vi "Refresh Access Codes.vi"(8 "error in":errorcluster, 9 "Refresh Token In":string, 11 "Authorization Code In":string) -> (0 "error out":errorcluster, 1 "Cluster":T1)   [LabVIEW 2016]
uses:
  <vilib>/httpClient/POSTBuffer.vi
  <vilib>/addons/_JKI.lib/Serialization/JSON/JKI JSON Serialization.lvlib
  <vilib>/httpClient/LabVIEWHTTPClient.lvlib
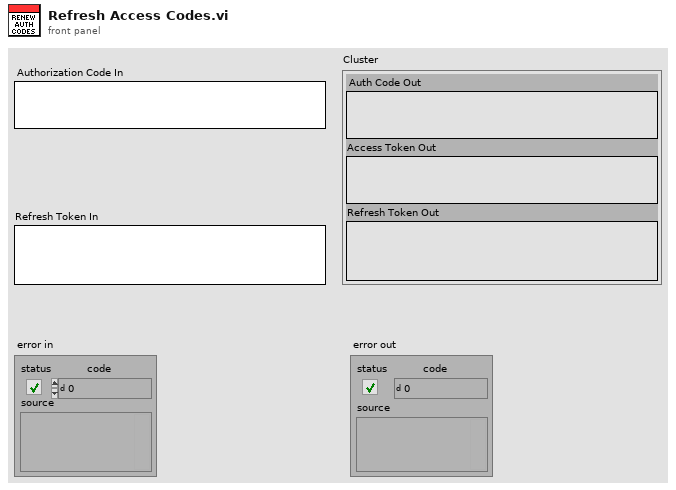
[diagram p1: front panel]
types:
  T1 = cluster{"Auth Code Out":string, "Access Token Out":string, "Refresh Token Out":string}
  T2 = cluster{"Access":string, "Refresh":string, "Authentication":string}
  T3 = cluster{"token_type":string, "scope":string, "access_token":string, "refresh_token":string, "user_id":string, "expires_in":i32}
  T4 = typedef "LabVIEWHTTPClient.lvlib/ClientHandle.ctl" = refnum<k1>
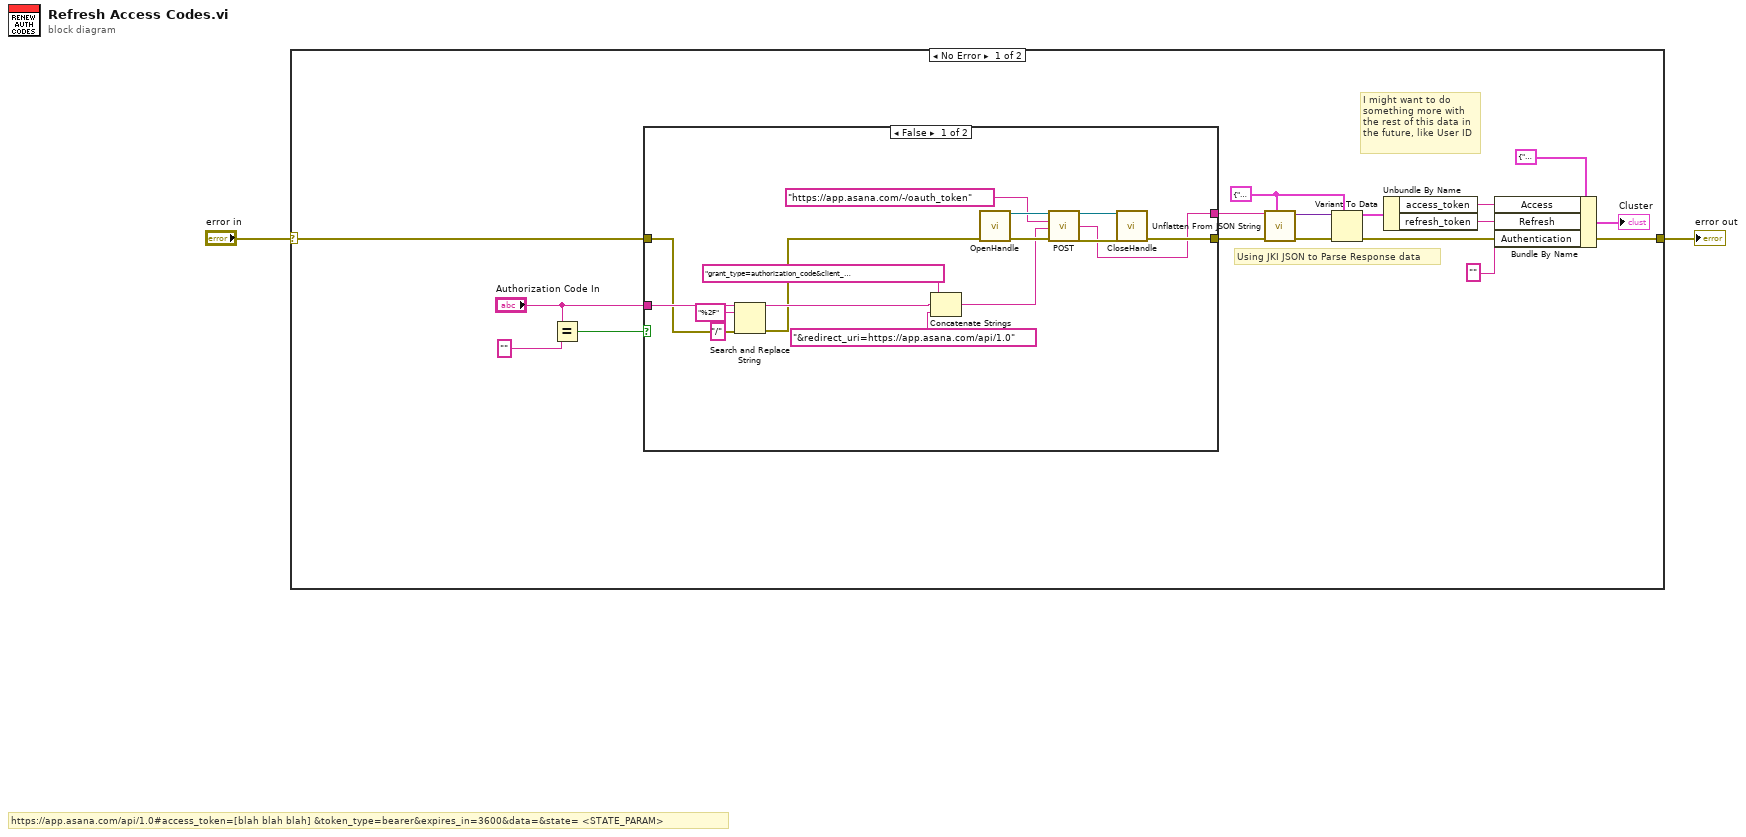
[diagram p0: block diagram]
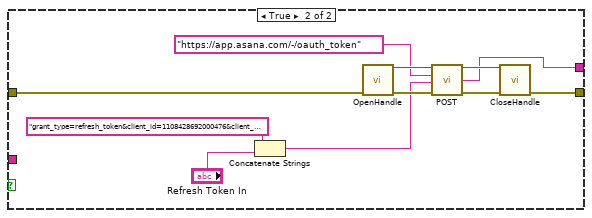
[diagram p2: hidden frame]
diagram:
  # "https://app.asana.com/api/1.0#access_token=[blah blah blah] &token_type=bearer&expires_in=3600&data=&state= <STATE_PARAM>"
  n1 = case shown="No Error" "error in" {
    selector: "error in" -> [w11 w46]
    tunnel: [w18 w46] -> w1
    frame No Error {
      w16 = T3 {"token_type"="", "scope"="", "access_token"="", "refresh_token"="", "user_id"="", "expires_in"=0}
      # "I might want to do something more with the rest of this data in the future, like User ID"
      # "Using JKI JSON to Parse Response data"
      n2 = Equal?(x="Authorization Code In", y="") -> (x = y?=w13:bool)
      n3 = case shown="False" w13 {
        tunnel: w11 -> [w22 w38]
        tunnel: [w31 w35] -> w10
        tunnel: [w25 w36] -> w8
        tunnel: "Authorization Code In" -> [w24 _]
        frame False {
          n4 = Search and Replace String(input string=w24, search string="%2F", replace string="/" ("replace string (\"\")"), error in=w22) -> (result string=w23:string, error out=w21:errorcluster)  [unwired: 4 in, 2 out]
          n5 = Concatenate Strings("grant_type=authorization_code&client_id=1108428692000476&client_secret=803bdca1138fccb00921b8f346728904&code=", w23, "&redirect_uri=https://app.asana.com/api/1.0") -> (w27:string)
          n6 = call <vilib>:"OpenHandle.vi"("error in (no error)"=w21) -> ("client handle out"=w30:T4, "error out"=w33:errorcluster)  [unwired: 13 in]
          n7 = call-poly <vilib>:"POST.vi"("client handle"=w30, "url"="https://app.asana.com/-/oauth_token", "buffer"=w27, "error in (no error)"=w33) -> ("client handle out"=w29:T4, "body"=w25:string, "error out"=w32:errorcluster)  [unwired: 8 in, 1 out]
          n8 = call <vilib>:"CloseHandle.vi"("client handle"=w29, "error in (no error)"=w32) -> ("error out"=w31:errorcluster)  [unwired: 13 in]
        }
        frame True {
          n9 = Concatenate Strings("grant_type=refresh_token&client_id=1108428692000476&client_secret=803bdca1138fccb00921b8f346728904&redirect_uri=https://app.asana.com/api/1.0&refresh_token=", "Refresh Token In") -> (w37:string)
          n10 = call <vilib>:"OpenHandle.vi"("error in (no error)"=w38) -> ("client handle out"=w41:T4, "error out"=w43:errorcluster)  [unwired: 13 in]
          n11 = call-poly <vilib>:"POST.vi"("client handle"=w41, "url"="https://app.asana.com/-/oauth_token", "buffer"=w37, "error in (no error)"=w43) -> ("client handle out"=w40:T4, "body"=w36:string, "error out"=w42:errorcluster)  [unwired: 8 in, 1 out]
          n12 = call <vilib>:"CloseHandle.vi"("client handle"=w40, "error in (no error)"=w42) -> ("error out"=w35:errorcluster)  [unwired: 13 in]
        }
      }
      n13 = call <vilib>:"Unflatten From JSON String.vi"("Type and Defaults"=w16, "error in (no error)"=w10, "JSON String"=w8) -> ("error out"=w17:errorcluster, "Variant"=w15:variant)  [unwired: 7 in]
      n14 = Variant To Data(error in=w17, type=w16, Variant=w15) -> (data=w14:T3, error out=w18:errorcluster)
      n15 = Unbundle By Name(w14) -> ("access_token"=w5:string, "refresh_token"=w4:string)
      n16 = Bundle By Name(cluster=T2 {"Access"="", "Refresh"="", "Authentication"=""}, "Access"=w5, "Refresh"=w4, "Authentication"="") -> (→"Cluster":T2)
    }
    frame Error {
    }
  }
  "error out" <- w1
